vi "A33ConfigurePRBS_py.vi"() -> ()   [LabVIEW 2022 SP3]
uses:
  <vilib>/addons/zeromq/zmq_socket.lvclass
panel:
  in  "Edge (4ns)":dbl=4e-09 format="%#_12g"
  in  "Sequenc type PN#":i32=7 min=3 max=32
  in  "Channel (1: Channel1)":i32(ring)=1 items=["Channel1"=1, "Channel2"=2]
  out "Standalone":bool
  out "socket out":refnum<class "zmq_socket.lvclass">
  in  "socket in":refnum<class "zmq_socket.lvclass">
  out "error out":errorcluster
  out "resulting string":string
  in  "Instrument":string="AG33600A_Gen1"
  in  "error in (no error)":errorcluster
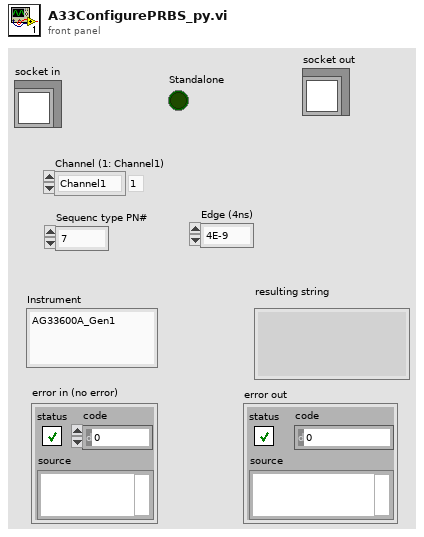
[diagram p1: front panel]
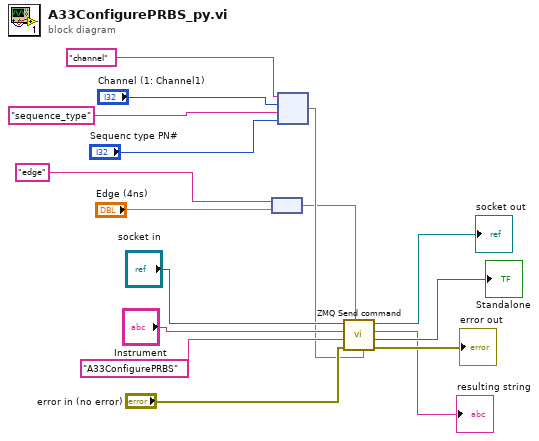
[diagram p0: block diagram]
diagram:
  n1 = node("edge" ("key"), "Edge (4ns)") -> (w1:map{string, dbl})
  n2 = node("channel" ("key"), "Channel (1: Channel1)", "sequence_type" ("key"), "Sequenc type PN#") -> (w2:map{string, i32})
  n3 = call "ZMQ Send command.vi"("Int args"=w2, "DBL args"=w1, "error in"="error in (no error)", "Command"="A33ConfigurePRBS", "Instrument"="Instrument", "socket in"="socket in") -> ("error out"=→"error out":errorcluster, "Standalone"=→"Standalone":bool, "Recieved message"=→"resulting string":string, "socket out"=→"socket out":refnum<class "zmq_socket.lvclass">)  [unwired: 2 in]
